vi "例程54-双机串行通信.vi"() -> ()   [LabVIEW 2016]
uses:
  <vilib>/Instr/_visa.llb/VISA Configure Serial Port (Instr).vi
panel:
  out "错误输出":errorcluster
  out "写返回数":u32
  out "读返回数":u32
  out "缓冲区":string
  in  "flow control (0:none)":u16(ring) caption="流控制（0:无）" items=["无", "XON/XOFF", "RTS/CTS", "XON/XOFF & RTS/CTS", "DTR/DSR", "XON/XOFF & DTR/DSR"]
  in  "stop bits (10: 1 bit)":u16(ring)=10 caption="停止位（10: 1位）" items=["1.0"=10, "1.5"=15, "2.0"=20]
  in  "parity (0:none)":enum16{"None", "Odd", "Even", "Mark", "Space"}(ring) caption="奇偶（0:无）"
  in  "Enable Termination\nChar (T)":bool=TRUE caption="启用终止符 (T)"
  in  "termination char\n(0xA = '\\n' = LF)":u8=10 caption="终止符\n(0xA = '\\n' = LF)" format="%.0x"
  in  "timeout (10sec)":u32=10000 caption="超时（10秒）"
  in  "data bits (8)":u16=8 caption="数据比特(8)" min=5 max=8 step=1
  in  "baud rate (9600)":u32=9600 caption="波特率(9600)"
  in  "VISA resource name":refnum<visa-resource-name> caption="VISA资源名称"
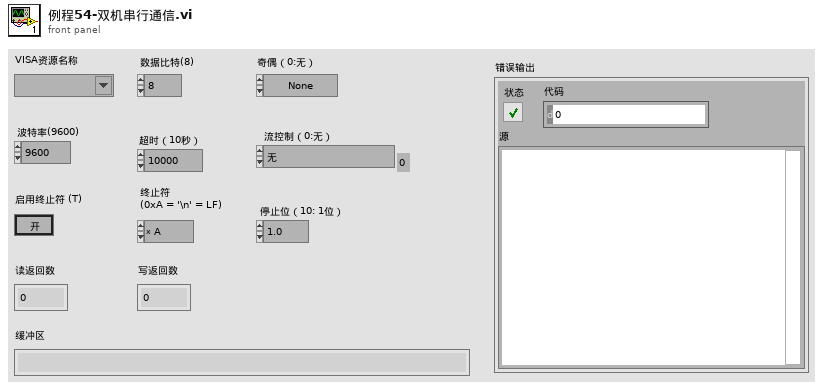
[diagram p1: front panel]
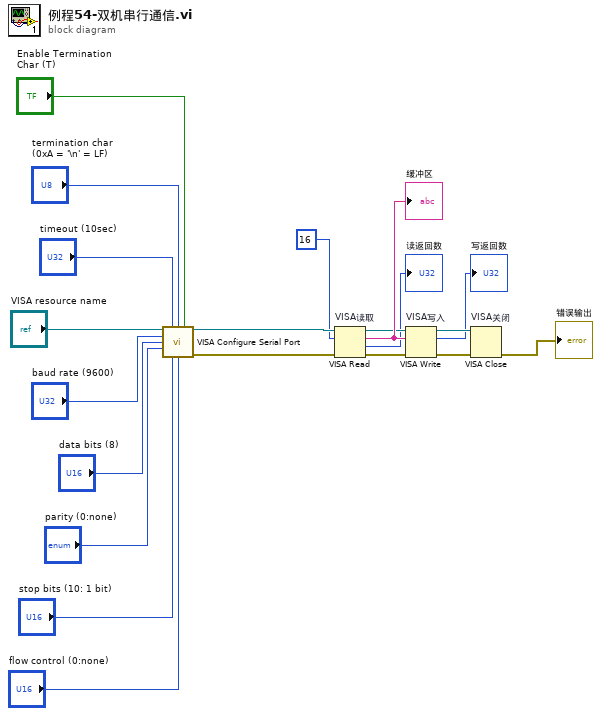
[diagram p0: block diagram]
diagram:
  n1 = call-poly "VISA Configure Serial Port"("VISA resource name"="VISA resource name", "timeout (10sec)"="timeout (10sec)", "termination char\n(0xA = '\\n' = LF)"="termination char\n(0xA = '\\n' = LF)", "Enable Termination\nChar (T)"="Enable Termination\nChar (T)", "baud rate (9600)"="baud rate (9600)", "data bits (8)"="data bits (8)", "parity (0:none)"="parity (0:none)", "stop bits (10: 1 bit)"="stop bits (10: 1 bit)", "flow control (0:none)"="flow control (0:none)") -> ("VISA resource name out"=w6:refnum<visa-resource-name>, "error out"=w5:errorcluster)  [unwired: 5 in]
  n2 = VISA Read "VISA读取"(VISA resource name=w6, byte count=u32 16 ("字节总数"), error in (no error)=w5) -> (VISA resource name out=w8:refnum<visa-resource-name>, read buffer=w9:string, return count=→"读返回数":u32, error out=w7:errorcluster)
  "缓冲区" <- w9
  n3 = VISA Write "VISA写入"(VISA resource name=w8, write buffer=w9, error in (no error)=w7) -> (VISA resource name out=w11:refnum<visa-resource-name>, return count=→"写返回数":u32, error out=w10:errorcluster)
  n4 = VISA Close "VISA关闭"(VISA resource name=w11, error in (no error)=w10) -> (error out=→"错误输出":errorcluster)
